vi "DefaultFromINI.vi"(8 "error in (no error)":errorcluster, 11 "NHRDCPower":refnum<class "NHRDCPower.lvclass">) -> (0 "error out":errorcluster, 3 "NHRDCPower":refnum<class "NHRDCPower.lvclass">)   [LabVIEW 2018, in "AcPwrPlugins.lvlib" / "NHRDCPower.lvclass"]
doc: "This VI reads the current configuration stored in the INI file."
uses:
  NHRDCPower.lvclass
  C:/Program Files (x86)/National Instruments/LabVIEW 2018/user.lib/NIST/BaseClasses/BasePlugin_class/BasePlugin.lvclass
  C:/Projects/ICDAS - Local tetsing/NistPluggableModules/AcPwr/AcPwrPlugins/AcPwrBaseClass/AcPwrBase.lvclass
  TypeDefs/Measurements.ctl
  TypeDefs/Device(s)Settings.ctl
  TypeDefs/Modules.ctl
  <userlib>/NIST/BaseClasses/BasePlugin_class/BasePlugin.lvclass/BasePlugin.ctl
  <userlib>/NIST/BaseClasses/BasePlugin_class/Accessors/Read PluginIniFilePath.vi
  AcPwrBaseClass/AcPwrBase.lvclass
  <vilib>/Utility/config.llb/NI_LVConfig.lvlib
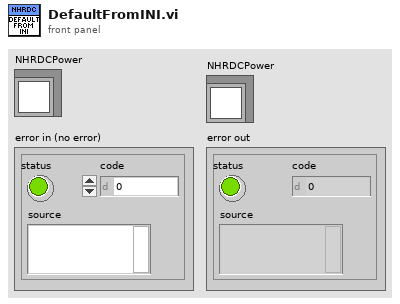
[diagram p1: front panel]
types:
  T1 = typedef "AcPwrPlugins.lvlib/NHRDCPower.lvclass/Device(s)Settings.ctl" = cluster{"MeasName":string, "Modules":T2}
  T2 = typedef "AcPwrPlugins.lvlib/NHRDCPower.lvclass/Modules.ctl" = cluster{"Handle":string, "Name":string, "id query (Yes)":bool, "reset device (Yes)":bool, "Connected":bool, "Initial Battery Detect Voltage (0)":dbl, "SafetySettings":cluster{"SetWatchDog?":bool, "Voltage (V)":dbl, "Current (A)":dbl, "Power (W)":dbl, "Voltage Delay (s)":dbl, "Current Delay (s)":dbl, "Power Delay (s)":dbl}, "Options String":string, "Aperture Time (s)":dbl, "operating state (Off)":i32, "OutputSettings":cluster{"Voltage (V)":dbl, "Current (A)":dbl, "Resistance (Ohms)":dbl, "Power (W)":dbl, "Enable Voltage":bool, "Enable Current":bool, "Enable Resistance":bool, "Enable Power":bool, "Macro After Step Delay  (s)":dbl, "Wait Value (V, A, W)":dbl, "Enable Wait":bool, "Wait on Value":i32}, "SlewRate":cluster{"Set Voltage Rate V/S":dbl, "Set Current Rate A/S":dbl, "Set Resistance Rate R/S":dbl, "Set Power Rate W/S":dbl}, "Macro":cluster{"Save Macro?":bool, "Load Macro From File?":bool, "Run Macro Continuously?":bool, "Use Macros?":bool, "Load Macro File Path":path, "Save Macro File Path":string}, "Regulation Gain (1=100%)":dbl, "UpdatingOntheFly":bool}[]
  T3 = typedef "AcPwrPlugins.lvlib/NHRDCPower.lvclass/Measurements.ctl" = cluster{"Handle":string, "Name":string, "Enabled":bool, "Measurement Value":sgl, "Measurement Type":enum16{"Power", "Current", "Voltage"}}[]
  T4 = typedef "NI_LVConfig.lvlib/Config Data RefNum.ctl" = refnum<k1>
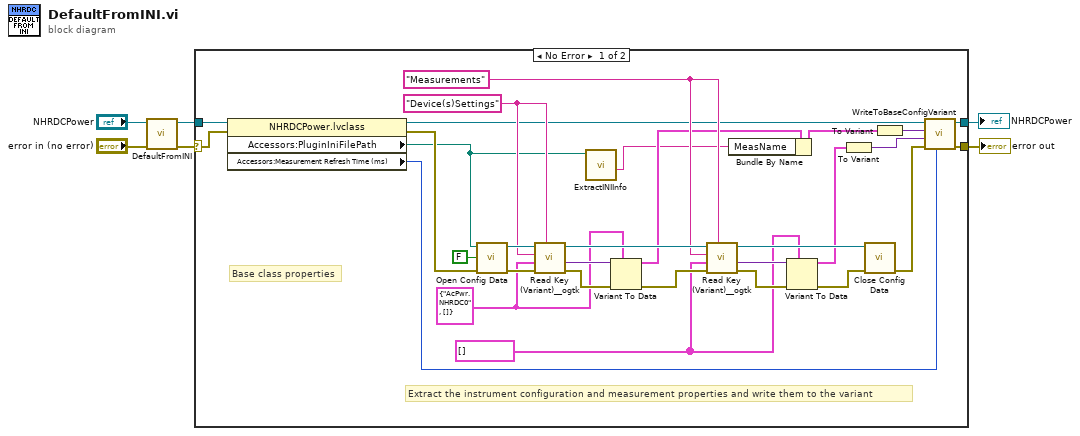
[diagram p0: block diagram]
diagram:
  n1 = call-parent "DefaultFromINI.vi"("error in (no error)"="error in (no error)", "AcPwrBase"="NHRDCPower") -> ("error out"=w6:errorcluster, "AcPwrBase"=w5:refnum<class "NHRDCPower.lvclass">)  [unwired: 8 in]
  n2 = case shown="No Error" w6 {
    selector: w6 -> [w11 w37]
    tunnel: w5 -> [w12 w38]
    tunnel: [w19 w38] -> w2
    tunnel: [w21 w37] -> w1
    frame No Error {
      w15 = T1 {"MeasName"="AcPwr.NHRDC0", "Modules"=[]} ("NHRDC")
      w22 = T3 [] ("Measurements")
      w23 = "Measurements" ("section")
      w31 = "Device(s)Settings" ("section")
      # "Extract the instrument configuration and measurement properties and write them to the variant"
      # "Base class properties"
      n3 = property class="NHRDCPower.lvclass"(reference=w12, error in=w11) -> (reference out=w16:refnum<class "NHRDCPower.lvclass">, error out=w30:errorcluster, "Accessors:PluginIniFilePath"=w9:path, "Accessors:Measurement Refresh Time (ms)"=w10:u32)
      n4 = call <vilib>:"Open Config Data.vi"("error in (no error)"=w30, "create file if necessary (T)"=FALSE, "configuration file path"=w9) -> ("error out"=w34:errorcluster, "refnum"=w35:T4)  [unwired: 6 in, 1 out]
      n5 = call <userlib>:"Read Key (Variant)__ogtk.vi"("section"=w31, "error in (no error)"=w34, "type"=w15, "key (optional)"=w31, "refnum"=w35) -> ("error out"=w32:errorcluster, "key-value"=w33:variant, "refnum out"=w27:T4)  [unwired: 3 in, 1 out]
      n6 = call "ExtractINIInfo.vi"("INI File Path"=w9) -> ("Plugin Name"=w7:string)  [unwired: 8 in, 2 out]
      n7 = Variant To Data(error in=w32, type=w15, Variant=w33) -> (data=w17:T1, error out=w24:errorcluster)
      n8 = call <userlib>:"Read Key (Variant)__ogtk.vi"("section"=w23, "error in (no error)"=w24, "type"=w22, "key (optional)"=w23, "refnum"=w27) -> ("error out"=w29:errorcluster, "key-value"=w28:variant, "refnum out"=w26:T4)  [unwired: 3 in, 1 out]
      n9 = Bundle By Name(cluster=w17, "MeasName"=w7) -> (w8:T1)
      n10 = Variant To Data(error in=w29, type=w22, Variant=w28) -> (data=w13:T3, error out=w25:errorcluster)
      n11 = To Variant(anything=w13) -> (Variant=w14:variant)
      n12 = call <vilib>:"Close Config Data.vi"("error in (no error)"=w25, "refnum"=w26) -> ("error out"=w20:errorcluster)  [unwired: 8 in, 1 out]
      n13 = To Variant(anything=w8) -> (Variant=w18:variant)
      n14 = call "WriteToBaseConfigVariant.vi"("Measurement Refresh Time (ms)"=w10, "error in (no error)"=w20, "Meas"=w14, "Config"=w18, "NHRDCPower in"=w16) -> ("error out"=w21:errorcluster, "NHRDCPower out"=w19:refnum<class "NHRDCPower.lvclass">)  [unwired: 5 in]
    }
    frame Error {
    }
  }
  "error out" <- w1
  "NHRDCPower" <- w2
